vi "pathplan_vertices.vi"(0 "目标位置（x,y）":dbl[](array[numeric]), 3 "当前位置":dbl[](array[numeric])) -> (8 "x":dbl[](array[numeric]), 9 "y":dbl[](array[numeric]))   [LabVIEW 2016]
uses:
  <vilib>/gmath/SpecialFunctions.llb/Factorial.vi
  <vilib>/imath/engines/lvmath2/RunTimeEngine/BuiltInFunctions/size/NIMS_I32Row=size(GRow).vi
  <instcachedir>/0/NIMS_I32Row=size(GRow)_E5C05C6B13124B29B774CC4F993D3C59.lvgen/NIMS_I32Row=size(GRow)_E5C05C6B13124B29B774CC4F993D3C59_001.vi
  <vilib>/imath/engines/lvmath2/RunTimeEngine/IndexRead/NIMS M(S,S).vi
  <instcachedir>/0/NIMS M(S,S)_AC51E74150A542F7991B9634C66F3096.lvgen/NIMS M(S,S)_AC51E74150A542F7991B9634C66F3096_002.vi
  <vilib>/imathl/engines/lvmath/Functions/Error Handling/Create Error.vi
  <vilib>/imath/engines/lvmath2/RunTimeEngine/BuiltInFunctions/int8/NIMS_int8(int).vi
  <instcachedir>/0/NIMS_int8(int)_D0907DA588884A6083B47B28B9C85019.lvgen/NIMS_int8(int)_D0907DA588884A6083B47B28B9C85019_000.vi
  <vilib>/imath/engines/lvmath2/RunTimeEngine/IndexRead/NIMS V(S).vi
  <instcachedir>/0/NIMS V(S)_0488751826AF41519A22953C041130DC.lvgen/NIMS V(S)_0488751826AF41519A22953C041130DC_000.vi
  <vilib>/imath/engines/lvmath2/RunTimeEngine/ErrorHandling/NIMS_Create Error From Enums.vi
  <vilib>/imath/engines/lvmath/Functions/Error Handling/MergeErrorsWrapper.vi
  <vilib>/imath/engines/lvmath2/RunTimeEngine/RangeToken/NIMS_Range_R2 - Integer.vi
  <instcachedir>/0/NIMS_Range_R2 - Integer_89B873E74E6E489885E44F751DD9C6BF.lvgen/NIMS_Range_R2 - Integer_89B873E74E6E489885E44F751DD9C6BF_000.vi
  <vilib>/imath/engines/lvmath2/RunTimeEngine/CommandStatement/MC_CommandStatement_break.vi
  <vilib>/imath/engines/lvmath2/RunTimeEngine/IndexRead/NIMS M($,S).vi
  <instcachedir>/0/NIMS M($,S)_3E5749BBB62E49528D4765A77F1F6D98.lvgen/NIMS M($,S)_3E5749BBB62E49528D4765A77F1F6D98_002.vi
  <vilib>/imath/engines/lvmath2/RunTimeEngine/ArithmeticOperatorToken/NIMS_ArithmeticOperator_minus.vi
  <instcachedir>/0/NIMS_ArithmeticOperator_minus_E3B65B1D26A44BB184AFDC5B3F458E3D.lvgen/NIMS_ArithmeticOperator_minus_E3B65B1D26A44BB184AFDC5B3F458E3D_003.vi
  <instcachedir>/0/NIMS_ArithmeticOperator_minus_E3B65B1D26A44BB184AFDC5B3F458E3D.lvgen/NIMS_ArithmeticOperator_minus_E3B65B1D26A44BB184AFDC5B3F458E3D_010.vi
  <vilib>/imath/engines/lvmath2/RunTimeEngine/BuiltInFunctions/abs/NIMS_abs(signed).vi
  <instcachedir>/0/NIMS_abs(signed)_C4FCB8E6058B49B797C7C8D53CA5F6EC.lvgen/NIMS_abs(signed)_C4FCB8E6058B49B797C7C8D53CA5F6EC_000.vi
  <vilib>/imath/engines/lvmath2/RunTimeEngine/RowToken/NIMS_RowToken_M_CV.vi
  <instcachedir>/0/NIMS_RowToken_M_CV_FA79F1D1D17D44459F3ED8E09EE8B625.lvgen/NIMS_RowToken_M_CV_FA79F1D1D17D44459F3ED8E09EE8B625_000.vi
  <vilib>/imath/engines/lvmath2/RunTimeEngine/IndexReplace/NIMS M($,S)=M.vi
  <instcachedir>/0/NIMS M($,S)=M_4ED09617E62F4BDFBC079C86D2836811.lvgen/NIMS M($,S)=M_4ED09617E62F4BDFBC079C86D2836811_000.vi
  <instcachedir>/0/NIMS V(S)_0488751826AF41519A22953C041130DC.lvgen/NIMS V(S)_0488751826AF41519A22953C041130DC_002.vi
  <vilib>/imath/engines/lvmath2/RunTimeEngine/IndexReplace/NIMS V(S)=S.vi
  <instcachedir>/0/NIMS V(S)=S_57E16554CB8B4B90AAB163894F717546.lvgen/NIMS V(S)=S_57E16554CB8B4B90AAB163894F717546_001.vi
  <instcachedir>/0/NIMS V(S)_0488751826AF41519A22953C041130DC.lvgen/NIMS V(S)_0488751826AF41519A22953C041130DC_003.vi
  <vilib>/imath/engines/lvmath2/RunTimeEngine/BuiltInFunctions/cos/NIMS_cos(C).vi
  <instcachedir>/0/NIMS_cos(C)_16E72F160CD540219ECD29F1B2AF26E5.lvgen/NIMS_cos(C)_16E72F160CD540219ECD29F1B2AF26E5_001.vi
  <instcachedir>/0/NIMS_abs(signed)_C4FCB8E6058B49B797C7C8D53CA5F6EC.lvgen/NIMS_abs(signed)_C4FCB8E6058B49B797C7C8D53CA5F6EC_002.vi
  <vilib>/imath/engines/lvmath2/RunTimeEngine/BuiltInFunctions/power/NIMS_power.vi
  <instcachedir>/0/NIMS_power_7E25183570944F38A5D8E4A9CE38EC54.lvgen/NIMS_power_7E25183570944F38A5D8E4A9CE38EC54_016.vi
  <vilib>/imath/engines/lvmath2/RunTimeEngine/BuiltInFunctions/max/2 inputs/NIMS_max(RG,RG)-no size check.vi
  <instcachedir>/0/NIMS_max(RG,RG)-no size check_F871939977644B7683C1350DCCAD7557.lvgen/NIMS_max(RG,RG)-no size check_F871939977644B7683C1350DCCAD7557_002.vi
  <vilib>/imath/engines/lvmath2/RunTimeEngine/BuiltInFunctions/min/2 inputs/NIMS_min(RG,RG)-no size check.vi
  <instcachedir>/0/NIMS_min(RG,RG)-no size check_7F67BAB91AFC452D9517D2EA1C8F5F88.lvgen/NIMS_min(RG,RG)-no size check_7F67BAB91AFC452D9517D2EA1C8F5F88_003.vi
  <vilib>/imath/engines/lvmath2/RunTimeEngine/VariableToken/NIMS_VariableToken_CondDefinedDefinedByReplace.vi
  <instcachedir>/0/NIMS_VariableToken_CondDefinedDefinedByReplace_D162CFFC24174562A9FEA619A91E1A56.lvgen/NIMS_VariableToken_CondDefinedDefinedByReplace_D162CFFC24174562A9FEA619A91E1A56_002.vi
  <instcachedir>/0/NIMS V(S)=S_57E16554CB8B4B90AAB163894F717546.lvgen/NIMS V(S)=S_57E16554CB8B4B90AAB163894F717546_003.vi
  <vilib>/imath/engines/lvmath2/RunTimeEngine/BuiltInFunctions/norm/NIMS_norm(GV,DBL).vi
  <instcachedir>/0/NIMS_norm(GV,DBL)_1268AFF3C646412B8C6EA3CE75D09042.lvgen/NIMS_norm(GV,DBL)_1268AFF3C646412B8C6EA3CE75D09042_000.vi
  <vilib>/imath/engines/lvmath2/RunTimeEngine/BuiltInFunctions/max/1 input/NIMS_max(RV).vi
  <instcachedir>/0/NIMS_max(RV)_237633DB1D604D5BA7001287DF3C7957.lvgen/NIMS_max(RV)_237633DB1D604D5BA7001287DF3C7957_002.vi
  <vilib>/imath/engines/lvmath2/RunTimeEngine/BuiltInFunctions/min/1 input/NIMS_min(RV).vi
  <instcachedir>/0/NIMS_min(RV)_EE2DD3E2888846108C5160A664B67832.lvgen/NIMS_min(RV)_EE2DD3E2888846108C5160A664B67832_002.vi
  <instcachedir>/0/NIMS_ArithmeticOperator_minus_E3B65B1D26A44BB184AFDC5B3F458E3D.lvgen/NIMS_ArithmeticOperator_minus_E3B65B1D26A44BB184AFDC5B3F458E3D_011.vi
  <vilib>/imath/engines/lvmath2/RunTimeEngine/MatrixToken/NIMS_MatrixToken_RV_RV.vi
  <instcachedir>/0/NIMS_MatrixToken_RV_RV_41289AEE7DB340EFBB9CA44FA48DA89B.lvgen/NIMS_MatrixToken_RV_RV_41289AEE7DB340EFBB9CA44FA48DA89B_002.vi
  <vilib>/imath/engines/lvmath2/RunTimeEngine/MatrixToken/NIMS_MatrixToken_M_RV.vi
  <instcachedir>/0/NIMS_MatrixToken_M_RV_EE14907D4B194E829889005D2F556E9C.lvgen/NIMS_MatrixToken_M_RV_EE14907D4B194E829889005D2F556E9C_001.vi
  <vilib>/imath/engines/lvmath2/RunTimeEngine/VariableToken/NIMS_VariableToken_CondDefined.vi
  <instcachedir>/0/NIMS_VariableToken_CondDefined_06E9DA95BD4D46A6BA55EC651A891960.lvgen/NIMS_VariableToken_CondDefined_06E9DA95BD4D46A6BA55EC651A891960_003.vi
  <vilib>/imath/engines/lvmath2/RunTimeEngine/IndexRead/NIMS V(V).vi
  <instcachedir>/0/NIMS V(V)_298D9CB7BFEB42B8BC8D9C3C28AE8C70.lvgen/NIMS V(V)_298D9CB7BFEB42B8BC8D9C3C28AE8C70_001.vi
  <vilib>/imath/engines/lvmath2/RunTimeSupport/NIMS_Get Scalar_w Error.vi
  <instcachedir>/0/NIMS_Get Scalar_w Error_59CA9FB130EE450F99234B5F2CCD930E.lvgen/NIMS_Get Scalar_w Error_59CA9FB130EE450F99234B5F2CCD930E_010.vi
  <instcachedir>/0/NIMS M(S,S)_AC51E74150A542F7991B9634C66F3096.lvgen/NIMS M(S,S)_AC51E74150A542F7991B9634C66F3096_000.vi
  <instcachedir>/0/NIMS_max(RG,RG)-no size check_F871939977644B7683C1350DCCAD7557.lvgen/NIMS_max(RG,RG)-no size check_F871939977644B7683C1350DCCAD7557_000.vi
  <instcachedir>/0/NIMS_min(RG,RG)-no size check_7F67BAB91AFC452D9517D2EA1C8F5F88.lvgen/NIMS_min(RG,RG)-no size check_7F67BAB91AFC452D9517D2EA1C8F5F88_001.vi
  <vilib>/imath/engines/lvmath2/RunTimeEngine/IndexReplace/NIMS M(S,S)=S.vi
  <instcachedir>/0/NIMS M(S,S)=S_98E40400474E4398B113AE20298B4F82.lvgen/NIMS M(S,S)=S_98E40400474E4398B113AE20298B4F82_000.vi
  <vilib>/imath/engines/lvmath2/RunTimeEngine/BuiltInFunctions/size/NIMS_I32=size(GM,I32).vi
  <instcachedir>/0/NIMS_I32=size(GM,I32)_122058B1B3294FAEA5DC209B92B394E4.lvgen/NIMS_I32=size(GM,I32)_122058B1B3294FAEA5DC209B92B394E4_004.vi
  <vilib>/imath/engines/lvmath2/RunTimeEngine/NodeEndStatement/NIMS_NodeEndStatement_Output.vi
  <instcachedir>/0/NIMS_NodeEndStatement_Output_53EC0D466D134D7ABD903AC30B43404B.lvgen/NIMS_NodeEndStatement_Output_53EC0D466D134D7ABD903AC30B43404B_005.vi
  <vilib>/imath/engines/lvmath2/RunTimeEngine/ErrorHandling/NIMS_Finalize Error.vi
  <vilib>/gmath/NI_Gmath.lvlib
panel:
  out "?":cluster{"Data_x":dbl[], "Data_y":dbl[]}(graph)
  out "?":cluster{"Data_x":dbl[], "Data_y":dbl[]}(graph)
  out "x/y":dbl[](array[numeric])
  out "?":cluster{"Data_x":dbl[], "Data_y":dbl[]}(graph)
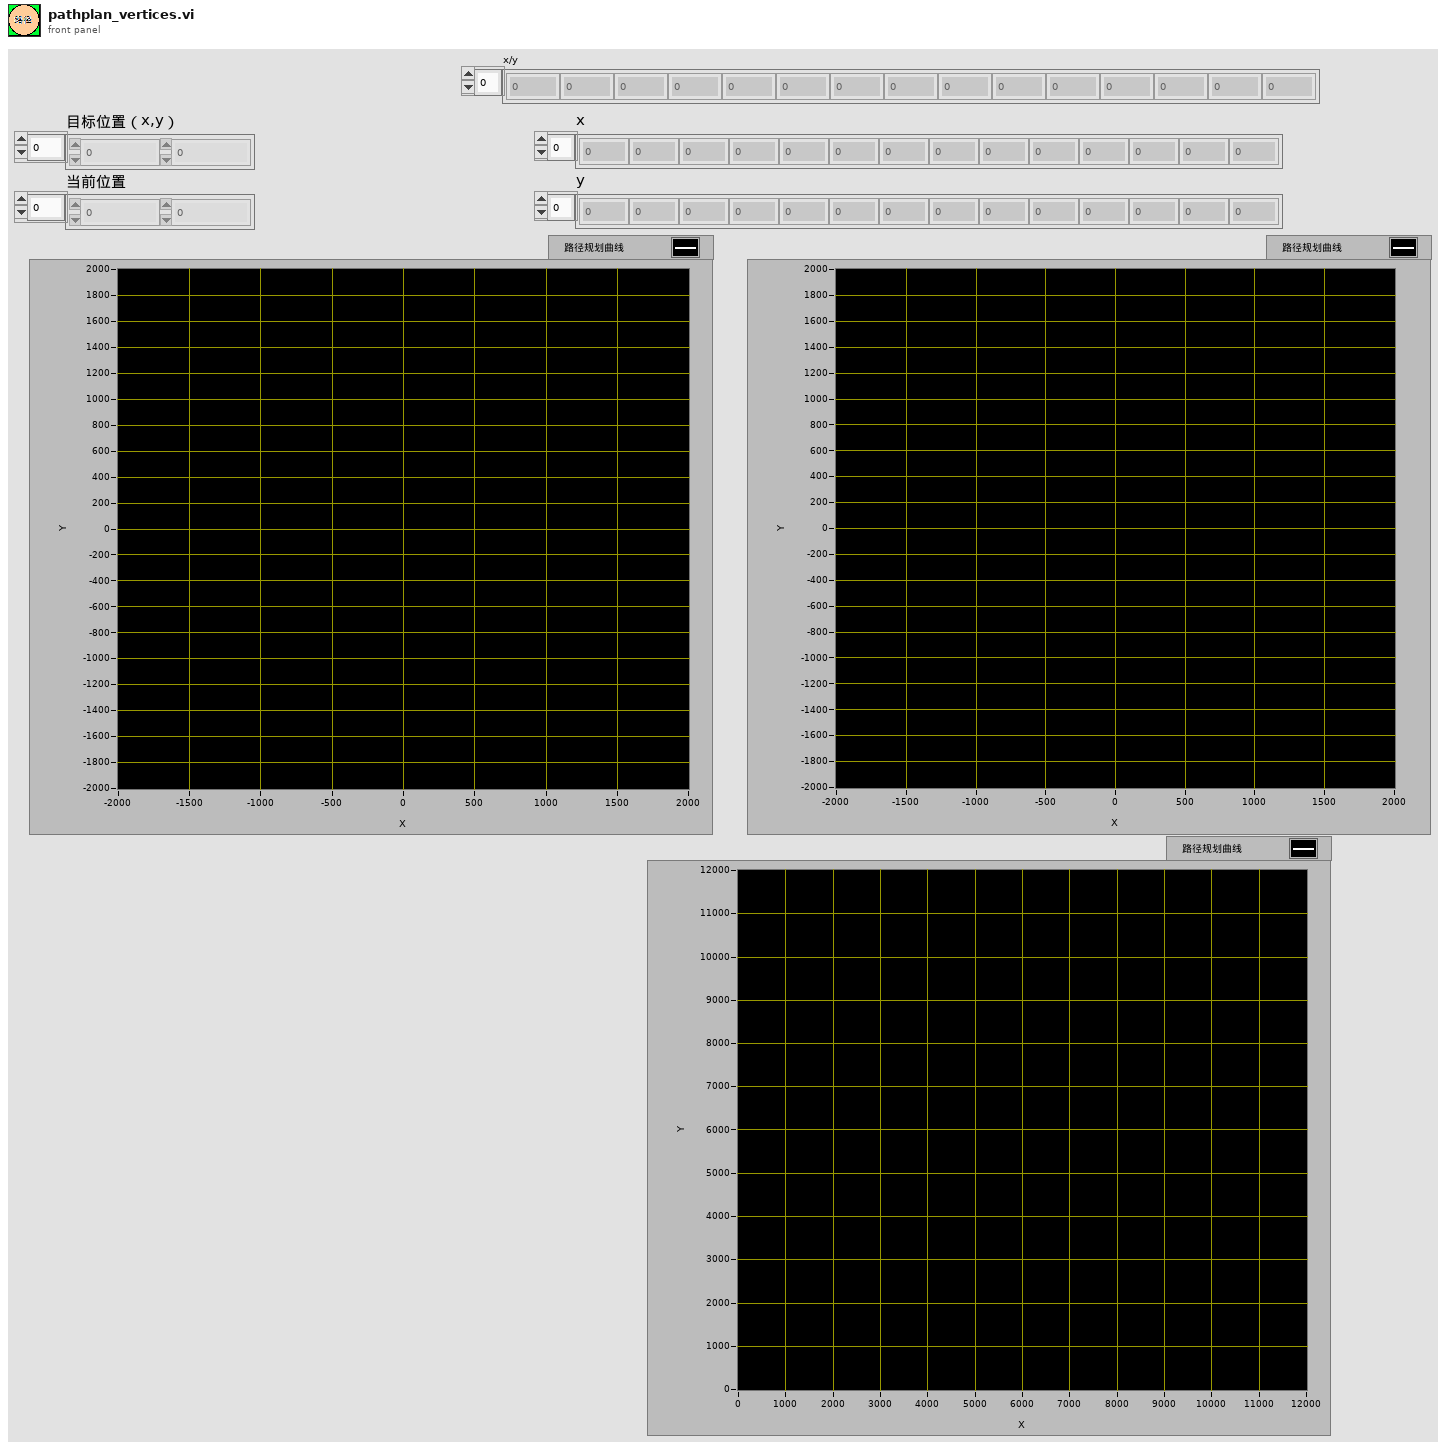
[diagram p1: front panel]
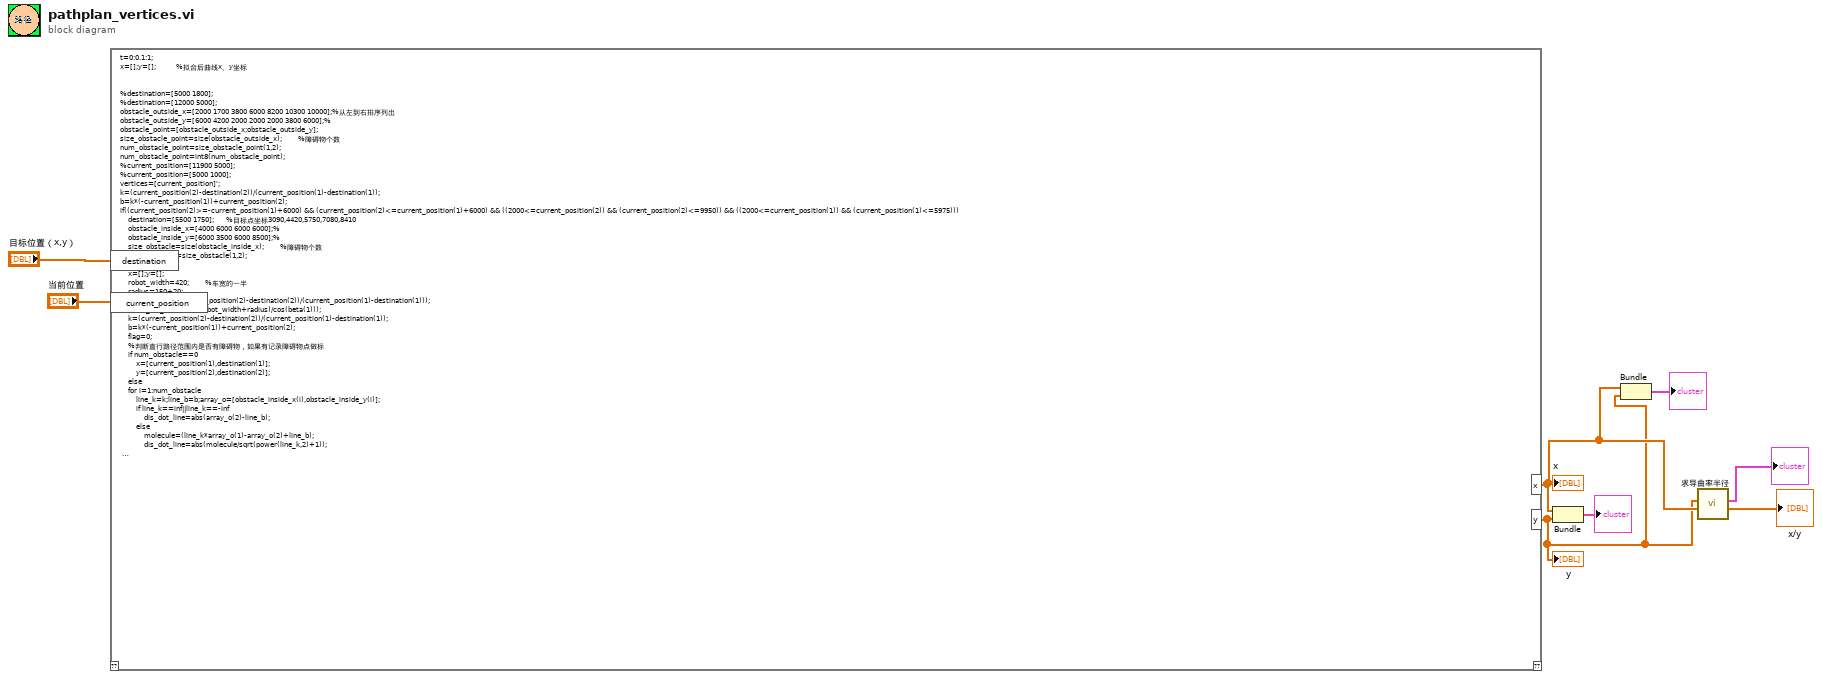
[diagram p0: block diagram]
diagram:
  n1 = mathscript code="t=0:0.1:1;\nx=[];y=[];          %拟合后曲线x、y坐标\n\n\n%destination=[5000 1800]; \n%destination=[12000 5000]; \nobstacle_outside_x=[2000 1700 3800 6000 8200 10300 10000];%从左到右排序列出\nobstacle_outside_y=[6000 4200 2000 2000 2000 3800 6000];%\nobstacle_point=[obstacle_outside_x;obstacle_outside_y];\nsize_obstacle_point=size(obstacle_outside_x);        %障碍物个数\nnum_obstacle_point=size_obstacle_point(1,2);\nnum_obstacle_point=int8(num_obstacle_point);\n%current_position=[11900 5000];\n%current_position=[5000 1000];\nvertices=[current_position]';\nk=(current_position(2)-destination(2))/(current_position(1)-destination(1));\nb=k*(-current_position(1))+current_position(2);\nif((current_position(2)>=-current_position(1)+6000) && (current_position(2)<=current_position(1)+6000) && ((2000<=current_position(2)) && (current_position(2)<=9950)) && ((2000<=current_position(1)) && (current_position(1)<=5975)))\n    destination=[5500 1750];      %目标点坐标3090,4420,5750,7080,8410\n    obstacle_inside_x=[4000 6000 6000 6000];%\n    obstacle_inside_y=[6000 3500 6000 8500];%\n    size_obstacle=size(obstacle_inside_x);        %障碍物个数\n    num_obstacle=size_obstacle(1,2);\n    count=0;\n    x=[];y=[];\n    robot_width=420;        %车宽的一半\n    radius=150+20;\n    beta(1)=atan((current_position(2)-destination(2))/(current_position(1)-destination(1)));\n    robot_dis_obs=abs((robot_width+radius)/cos(beta(1)));\n    k=(current_position(2)-destination(2))/(current_position(1)-destination(1));\n    b=k*(-current_position(1))+current_position(2);\n    flag=0;\n    %判断直行路径范围内是否有障碍物，如果有记录障碍物点做标\n    if num_obstacle==0\n        x=[current_position(1),destination(1)];\n        y=[current_position(2),destination(2)];\n    else\n    for i=1:num_obstacle\n        line_k=k;line_b=b;array_o=[obstacle_inside_x(i),obstacle_inside_y(i)];\n        if line_k==inf||line_k==-inf\n            dis_dot_line=abs(array_o(2)-line_b);\n        else\n            molecule=(line_k*array_o(1)-array_o(2)+line_b);\n            dis_dot_line=abs(molecule/sqrt(power(line_k,2)+1));\n        end\n%         dis_line=dot_line(k,b,[obstacle_inside_x(i),obstacle_inside_y(i)]);\n        dis_line=dis_dot_line;\n        if (dis_line<robot_width+radius || dis_line==robot_width+radius)&&(obstacle_inside_x(i)<max(destination(1),current_position(1))+robot_width+radius&&obstacle_inside_x(i)>min(destination(1),current_position(1))-robot_width+radius&&obstacle_inside_y(i)<max(destination(2),current_position(2))+robot_width+radius&&obstacle_inside_y(i)>min(destination(2),current_position(2))-robot_width+radius)\n            in_obstacle(count+1)=obstacle_inside_x(i);\n            in_obstacle(count+2)=obstacle_inside_y(i);\n            count=count+2;\n        end\n    end\n    cosalph=(current_position(1)-destination(1))/norm(destination-current_position);\n    sinalph=(current_position(2)-destination(2))/norm(destination-current_position);\n    if current_position(1)<destination(1)\n        cosalph=-cosalph;\n        sinalph=-sinalph;\n    end\n        if (count==0)       %(k==inf||k==-inf)||\n            x=[current_position(1),destination(1)];\n            y=[current_position(2),destination(2)];\n        else\n            %关于障碍物点x、y轴的偏移量\n            x_offset=(robot_width+radius);\n            y_offset=(robot_width+radius);\n            %旋转坐标系下的偏移量\n            acos=x_offset*cosalph;asin=x_offset*sinalph;\n            bcos=y_offset*cosalph;bsin=y_offset*sinalph;\n\n            if count==2 %一个障碍物\n                %当障碍物在两点连线上方时\n                if (in_obstacle(2)>(k*in_obstacle(1)+b))||(k==inf&&destination(1)>obstacle_inside_x(i))\n                    %先进行选取四点坐标\n                    temp_position1=[in_obstacle(1)+acos+bsin,in_obstacle(2)+asin-bcos];\n                    temp_position2=[in_obstacle(1)-acos+bsin,in_obstacle(2)-asin-bcos];\n                    if current_position(1)>destination(1)\n                        if temp_position1(1)>temp_position2(1)\n                            vertices=[current_position;temp_position1;temp_position2;destination]';\n                        else\n                            vertices=[current_position;temp_position2;temp_position1;destination]';\n                        end\n                    else\n                        if temp_position1(1)>temp_position2(1)\n                            vertices=[current_position;temp_position2;temp_position1;destination]';\n                        else\n                            vertices=[current_position;temp_position1;temp_position2;destination]';\n                        end\n                    end\n                else\n                    temp_position1=[in_obstacle(1)+acos-bsin,in_obstacle(2)+asin+bcos];\n                    temp_position2=[in_obstacle(1)-acos-bsin,in_obstacle(2)-asin+bcos];\n                    if current_position(1)>destination(1)\n                        if temp_position1(1)>temp_position2(1)\n                            vertices=[current_position;temp_position1;temp_position2;destination]';\n                        else\n                            vertices=[current_position;temp_position2;temp_position1;destination]';\n                        end\n                    else\n                        if temp_position1(1)>temp_position2(1)\n                            vertices=[current_position;temp_position2;temp_position1;destination]';\n                        else\n                            vertices=[current_position;temp_position1;temp_position2;destination]';\n                        end\n                    end\n                    for i=1:num_obstacle\n                         if (obstacle_inside_x(i)~=in_obstacle(1))&&(obstacle_inside_x(i)<max(vertices(1,1),vertices(1,2))&&obstacle_inside_x(i)>min(vertices(1,1),vertices(1,2)))&&(obstacle_inside_y(i)<((vertices(2,2)-vertices(2,1))/(vertices(1,2)-vertices(1,1))*obstacle_inside_x(i)+vertices(2,2)-(vertices(2,2)-vertices(2,1))/(vertices(1,2)-vertices(1,1))*vertices(1,2)+robot_dis_obs))&&(obstacle_inside_y(i)>((vertices(2,2)-vertices(2,1))/(vertices(1,2)-vertices(1,1))*obstacle_inside_x(i)+vertices(2,2)-(vertices(2,2)-vertices(2,1))/(vertices(1,2)-vertices(1,1))*vertices(1,2)-robot_dis_obs))||(obstacle_inside_x(i)~=in_obstacle(1))&&(obstacle_inside_x(i)<max(vertices(1,3),vertices(1,4))&&obstacle_inside_x(i)>min(vertices(1,3),vertices(1,4)))&&(obstacle_inside_y(i)<((vertices(2,4)-vertices(2,3))/(vertices(1,4)-vertices(1,3))*obstacle_inside_x(i)+vertices(2,4)-(vertices(2,4)-vertices(2,3))/(vertices(1,4)-vertices(1,3))*vertices(1,4)+robot_dis_obs))&&(obstacle_inside_y(i)>((vertices(2,4)-vertices(2,3))/(vertices(1,4)-vertices(1,3))*obstacle_inside_x(i)+vertices(2,4)-(vertices(2,4)-vertices(2,3))/(vertices(1,4)-vertices(1,3))*vertices(1,4)-robot_dis_obs))\n                            in_obstacle(count+1)=obstacle_inside_x(i);\n                            in_obstacle(count+2)=obstacle_inside_y(i);\n                            count=count+2;\n                            break;\n                        end\n                    end\n                end\n            else\n                if k*max(obstacle_inside_x)+b<min(obstacle_inside_y)\n                    temp_position1=[max(obstacle_inside_x)+x_offset,min(obstacle_inside_y)+y_offset];\n                    temp_position2=[max(obstacle_inside_x)-x_offset,min(obstacle_inside_y)+y_offset];\n                    if norm(current_position-temp_position1)<norm(current_position-temp_position2)\n                        temp1=temp_position1;\n                        temp2=temp_position2;\n                    else\n                        temp1=temp_position2;\n                        temp2=temp_position1;\n                    end\n                    vertices=[current_position;temp1;temp2;destination]';\n                else\n                    temp_position1=[max(obstacle_inside_x)+x_offset,max(obstacle_inside_y)-y_offset];\n                    temp_position2=[max(obstacle_inside_x)-x_offset,max(obstacle_inside_y)-y_offset];\n                    if norm(current_position-temp_position1)<norm(current_position-temp_position2)\n                        temp1=temp_position1;\n                        temp2=temp_position2;\n                    else\n                        temp1=temp_position2;\n                        temp2=temp_position1;\n                    end\n                    vertices=[current_position;temp1;temp2;destination]';\n                end\n            end\n            if count==4%两个障碍物\n                %当两个都在直线上方时\n                if (in_obstacle(2)>(k*in_obstacle(1)+b)||in_obstacle(2)==(k*in_obstacle(1)+b))&&(in_obstacle(4)>(k*in_obstacle(3)+b)||in_obstacle(4)==(k*in_obstacle(3)+b))\n                    temp_position1=[in_obstacle(1)+acos+bsin,in_obstacle(2)+asin-bcos];\n                    temp_position2=[in_obstacle(1)-acos+bsin,in_obstacle(2)-asin-bcos];\n                    temp_position3=[in_obstacle(3)+acos+bsin,in_obstacle(4)+asin-bcos];\n                    temp_position4=[in_obstacle(3)-acos+bsin,in_obstacle(4)-asin-bcos];\n                    flag=1;\n                    if norm(current_position-[in_obstacle(1),in_obstacle(2)])<norm(current_position-[in_obstacle(3),in_obstacle(4)])\n                        if norm(current_position-temp_position1)<norm(current_position-temp_position2)\n                            temp1=temp_position1;\n                            temp2=temp_position2;\n                        else\n                            temp1=temp_position2;\n                            temp2=temp_position1;\n                        end\n                        if norm(destination-temp_position3)<norm(destination-temp_position4)\n                            temp3=temp_position4;\n                            temp4=temp_position3;\n                        else\n                            temp3=temp_position3;\n                            temp4=temp_position4;\n                        end\n                    else\n                        if norm(current_position-temp_position3)<norm(current_position-temp_position4)\n                            temp1=temp_position3;\n                            temp2=temp_position4;\n                        else\n                            temp1=temp_position4;\n                            temp2=temp_position3;\n                        end\n                        if norm(destination-temp_position1)<norm(destination-temp_position2)\n                            temp3=temp_position2;\n                            temp4=temp_position1;\n                        else\n                            temp3=temp_position1;\n                            temp4=temp_position2;\n                        end\n                    end\n                    vertices=[current_position;temp1;temp4;destination ]';\n                    %当右侧的在直线下方，左侧的在直线上方\n                elseif in_obstacle(2)<(k*in_obstacle(1)+b)&&in_obstacle(4)>(k*in_obstacle(3)+b)\n                    temp_position1=[in_obstacle(1)+acos-bsin,in_obstacle(2)+asin+bcos];\n                    temp_position2=[in_obstacle(1)-acos-bsin,in_obstacle(2)-asin+bcos];\n                    temp_position3=[in_obstacle(3)+acos+bsin,in_obstacle(4)+asin-bcos];\n                    temp_position4=[in_obstacle(3)-acos+bsin,in_obstacle(4)-asin-bcos];\n                    if norm(current_position-[in_obstacle(1),in_obstacle(2)])<norm(current_position-[in_obstacle(3),in_obstacle(4)])\n                        if norm(current_position-temp_position1)<norm(current_position-temp_position2)\n                            temp1=temp_position1;\n                            temp2=temp_position2;\n                        else\n                            temp1=temp_position2;\n                            temp2=temp_position1;\n                        end\n                        if norm(destination-temp_position3)<norm(destination-temp_position4)\n                            temp3=temp_position4;\n                            temp4=temp_position3;\n                        else\n                            temp3=temp_position3;\n                            temp4=temp_position4;\n                        end\n                    else\n                        if norm(current_position-temp_position3)<norm(current_position-temp_position4)\n                            temp1=temp_position3;\n                            temp2=temp_position4;\n                        else\n                            temp1=temp_position4;\n                            temp2=temp_position3;\n                        end\n                        if norm(destination-temp_position1)<norm(destination-temp_position2)\n                            temp3=temp_position2;\n                            temp4=temp_position1;\n                        else\n                            temp3=temp_position1;\n                            temp4=temp_position2;\n                        end\n                    end\n                    vertices=[current_position;temp1;temp2;temp3;temp4;destination ]';\n                else%当两点都在直线下方时\n                    temp_position1=[in_obstacle(1)+acos-bsin,in_obstacle(2)+asin+bcos];\n                    temp_position2=[in_obstacle(1)-acos-bsin,in_obstacle(2)-asin+bcos];\n                    temp_position3=[in_obstacle(3)+acos-bsin,in_obstacle(4)+asin+bcos];\n                    temp_position4=[in_obstacle(3)-acos-bsin,in_obstacle(4)-asin+bcos];\n                    if norm(current_position-[in_obstacle(1),in_obstacle(2)])<norm(current_position-[in_obstacle(3),in_obstacle(4)])\n                        if norm(current_position-temp_position1)<norm(current_position-temp_position2)\n                            temp1=temp_position1;\n                            temp2=temp_position2;\n                        else\n                            temp1=temp_position2;\n                            temp2=temp_position1;\n                        end\n                        if norm(destination-temp_position3)<norm(destination-temp_position4)\n                            temp3=temp_position4;\n                            temp4=temp_position3;\n                        else\n                            temp3=temp_position3;\n                            temp4=temp_position4;\n                        end\n                    else\n                        if norm(current_position-temp_position3)<norm(current_position-temp_position4)\n                            temp1=temp_position3;\n                            temp2=temp_position4;\n                        else\n                            temp1=temp_position4;\n                            temp2=temp_position3;\n                        end\n                        if norm(destination-temp_position1)<norm(destination-temp_position2)\n                            temp3=temp_position2;\n                            temp4=temp_position1;\n                        else\n                            temp3=temp_position1;\n                            temp4=temp_position2;\n                        end\n                    end\n                    vertices=[current_position;temp1;temp4;destination ]';\n                end\n            end\n            if count==6\n            %当三个都在直线下方时\n                temp_position1=[in_obstacle(1)+acos-bsin,in_obstacle(2)+asin+bcos];\n                temp_position2=[in_obstacle(1)-acos-bsin,in_obstacle(2)-asin+bcos];\n                temp_position3=[in_obstacle(3)+acos-bsin,in_obstacle(4)+asin+bcos];\n                temp_position4=[in_obstacle(3)-acos-bsin,in_obstacle(4)-asin+bcos];\n                temp_position5=[in_obstacle(5)+acos-bsin,in_obstacle(6)+asin+bcos];\n                temp_position6=[in_obstacle(5)-acos-bsin,in_obstacle(6)-asin+bcos];\n                vertices  = [current_position;temp_position5;temp_position6;temp_position3;temp_position4;temp_position1;temp_position2;destination]';\n                if(current_position(2)<in_obstacle(end))\n                    vertices(:,2)=[];\n                end\n            end\n            if(current_position(2)<in_obstacle(end))                   \n                vertices(:,(end-2))=[];\n            end\n            vertices(2,2)=vertices(2,2)-1.5*radius;\n        end\n    end\nelse %在外部运行的情况\n    flag_change1=0;\n    flag_change2=0;\n    for i=1:num_obstacle_point-1\n        A=current_position;B=destination;C=obstacle_point(:,i)';D=obstacle_point(:,i+1)';\n        flag_intersect=0;\n        AB=B-A;\n        AC=C-A;\n        AD=D-A;\n        AB_cross_AC=AB(1)*AC(2)-AC(1)*AB(2);\n        AB_cross_AC=AB_cross_AC/abs(AB_cross_AC);\n        AB_cross_AD=AB(1)*AD(2)-AD(1)*AB(2);\n        AB_cross_AD=AB_cross_AD/abs(AB_cross_AD);\n        if (AB_cross_AC*AB_cross_AD<=0)\n            flag_intersect=1;\n        end         \n        if flag_intersect==1\n            if(current_position(1)<destination(1))\n                current_position=obstacle_point(:,i+1)'-[0,500];\n                vertices=[vertices,current_position'];\n                flag_change1=1;\n            else\n                destination=obstacle_point(:,i+1)'-[0,500];\n                vertices=[vertices,destination'];\n                flag_change2=1;\n                if(i==num_obstacle_point-2)\n                    vertices(:,1)=[];\n                    vertices=[vertices,current_position'];         \n                end\n            end\n        end\n    end\n    if(flag_change1==1)\n        vertices=[vertices,destination'];\n    end\n    if(flag_change2==1)\n        vertices(:,1)=[];\n        vertices=[vertices,current_position'];\n    end\nend\n\n\n%贝塞尔曲线拟合\nNumPoint=size(vertices,2)-1;\nx=(1-t).^(NumPoint)*vertices(1,1);\ny=(1-t).^(NumPoint)*vertices(2,1);\nfor j=1:NumPoint\n    w=factorial(NumPoint)/(factorial(j)*factorial(NumPoint-j))*(1-t).^(NumPoint-j).*t.^(j);\n    x=x+w*vertices(1,j+1);\n    y=y+w*vertices(2,j+1);\nend"("destination"="目标位置（x,y）", "current_position"="当前位置") -> ("x"=w2:dbl[], "y"=w1:dbl[])  [unwired: 1 in, 1 out]
  "x" <- w2
  "y" <- w1
  n2 = Bundle("x"=w2, "y"=w1) -> (→"?":cluster{"x":dbl[], "y":dbl[]})  [unwired: 1 in]
  n3 = Bundle("x"=w2, "y"=w1) -> (→"?":cluster{"x":dbl[], "y":dbl[]})  [unwired: 1 in]
  n4 = call "求导曲率半径.vi"("x"=w2, "y"=w1) -> ("x/y"=→"x/y":dbl[], 2:→"?":cluster{"Data_x":dbl[], "Data_y":dbl[]})  [unwired: 8 in]
